vi "ExcelRead.vi"(9 "Count":cluster{"Sheet":i32, "Row":i32, "Column":i32}={"Sheet"=5, "Row"=128, "Column"=5}, 10 "Start Position":cluster{"Sheet":i32, "Row":i32, "Column":i32}={"Sheet"=0, "Row"=2, "Column"=1}, 11 "File Name":path) -> (2 "Sheets Name":string[](array[string]), 3 "Values":string[][][](array[string]))   [LabVIEW 2014]
uses:
  Data/Polymorphic VIs/Get Cell (String).vi
  Data/Polymorphic VIs/Get Cell (DBL).vi
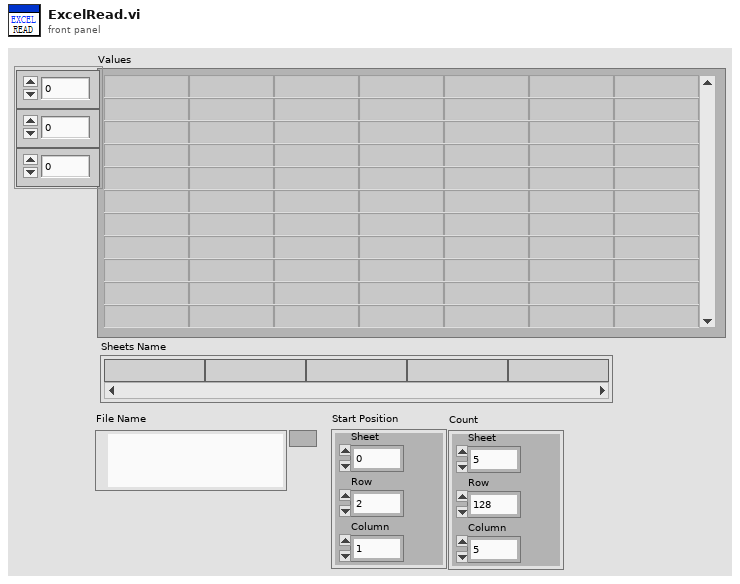
[diagram p1: front panel]
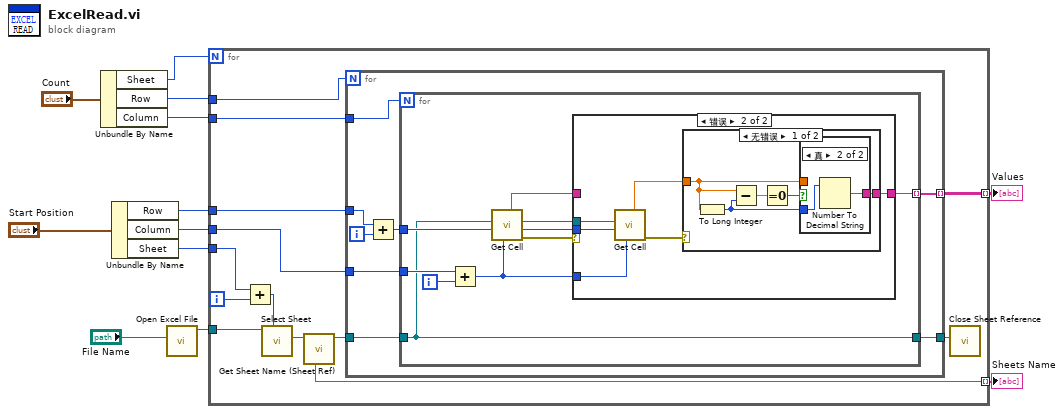
[diagram p0: block diagram]
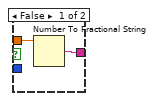
[diagram p3: hidden frame]
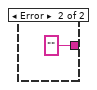
[diagram p4: hidden frame]
diagram:
  n1 = Unbundle By Name("Count") -> ("Sheet"=w7:i32, "Row"=w6:i32, "Column"=w5:i32)
  n2 = Unbundle By Name("Start Position") -> ("Row"=w1:i32, "Column"=w2:i32, "Sheet"=w3:i32)
  n3 = call "Open Excel File.vi"("File Name"="File Name") -> ("IWorkbook Reference Out"=w12:refnum<k24>)  [unwired: 9 in, 1 out]
  n4 = for {
    N: w7 -> [_]
    tunnel: w12 -> [w25]
    tunnel: [w23] -> w11 mode=indexing
    tunnel: [w21] -> w10 mode=indexing
    tunnel: w6 -> [w20]
    tunnel: w5 -> [w19]
    tunnel: w3 -> [w17]
    tunnel: w2 -> [w15]
    tunnel: w1 -> [w14]
    i -> [w18]
    n5 = Add(x=w17, y=w18) -> (x+y=w16:i32)
    n6 = call "Select Sheet.vi"("Sheet (0)"=w16, "IWorkbook Reference"=w25) -> ("Sheet Reference"=w24:refnum<k24>)  [unwired: 7 in, 2 out]
    n7 = call "Get Sheet Name (Sheet Ref).vi"("Sheet Reference"=w24) -> ("Sheet Reference out"=w22:refnum<k24>, "Sheet Name (Sheet1)"=w23:string)  [unwired: 8 in, 1 out]
    n8 = for {
      N: w20 -> [_]
      tunnel: w22 -> [w33]
      tunnel: [w32] -> w21 mode=indexing
      tunnel: w19 -> [w31]
      tunnel: w15 -> [w30]
      tunnel: w14 -> [w29]
      tunnel: [w26] -> w13
      i -> [w28]
      n9 = Add(x=w29, y=w28) -> (x+y=w27:i32)
      n10 = for {
        N: w31 -> [_]
        tunnel: w33 -> [w34]
        tunnel: w27 -> [w38]
        tunnel: [w39] -> w32 mode=indexing
        tunnel: w30 -> [w35]
        tunnel: [w34] -> w26
        i -> [w36]
        n11 = Add(x=w35, y=w36) -> (x+y=w37:i32)
        n12 = call-poly "Get Cell.vi"("Column"=w37, "Row"=w38, "Sheet Reference"=w34) -> ("error out"=w42:errorcluster, "Sheet Reference out"=w41:refnum<k24>, "Value"=w40:string)  [unwired: 6 in]
        n13 = case shown="错误" w42 {
          tunnel: w41 -> [_ w49]
          tunnel: w40 -> [w43 _]
          tunnel: [w43 w48] -> w39
          tunnel: w38 -> [_ w45]
          tunnel: w37 -> [_ w46]
          frame No Error {
          }
          frame Error {
            n14 = call-poly "Get Cell.vi"("Column"=w46, "Row"=w45, "Sheet Reference"=w49) -> ("error out"=w44:errorcluster, "Value"=w47:dbl)  [unwired: 6 in, 1 out]
            n15 = case shown="无错误" w44 {
              tunnel: [w53 ""] -> w48
              tunnel: w47 -> [w50 _]
              frame No Error {
                n16 = To Long Integer(number=w50) -> (32bit integer=w52:i32)
                n17 = Subtract(x=w50, y=w52) -> (x-y=w54:dbl)
                n18 = Equal To 0?(x=w54) -> (x = 0?=w51:bool)
                n19 = case shown="真" w51 {
                  tunnel: [w55 w58] -> w53
                  tunnel: w52 -> [_ w57]
                  tunnel: w50 -> [w56 _]
                  frame False {
                    n20 = Number To Fractional String(number=w56) -> (F-format string=w55:string)  [unwired: 3 in]
                  }
                  frame True {
                    n21 = Number To Decimal String(number=w57) -> (decimal integer string=w58:string)  [unwired: 1 in]
                  }
                }
              }
              frame Error {
              }
            }
          }
        }
      }
    }
    n22 = call "Close Sheet Reference.vi"("Sheet Reference"=w13) -> ()  [unwired: 10 in, 1 out]
  }
  "Sheets Name" <- w11
  "Values" <- w10
